vi "UpdateAcquisitionStats.vi"(8 "error in (no error)":errorcluster, 11 "configuration":T1 {"FixedSizeX31"."InputConfig" items=["AC Coupled", "DC Coupled", "IEPE AC Coupled"]}) -> (0 "error out":errorcluster, 2 "settling time requirement met?":bool, 3 "configuration":T1 {"FixedSizeX31"."InputConfig" items=["AC Coupled", "DC Coupled", "IEPE AC Coupled"]})   [LabVIEW 2017, in "McsaFpgaAcquisition.lvlib"]
uses:
  <vilib>/addons/InsightCM/Devices/Shared/Mcsa/McsaFpgaAcquisition/McsaFpgaAcquisition.lvlib
  <vilib>/addons/InsightCM/Devices/Shared/Mcsa/McsaFpgaAcquisition/controls/Configuration.ctl
  <vilib>/addons/InsightCM/Devices/Shared/Cms/CmsAcquisition/controls/FixedSizeArrays.ctl
  <vilib>/LabVIEW Targets/FPGA/cRIO/shared/nicrio_ModuleControls/nicrio_cRIO-9232_ConfigModeRing.ctl
  <vilib>/addons/InsightCM/Devices/Shared/Cms/cRIOWfmAcq/subVIs/RIO Wfm Cust Ctrls/rwfm_SamplingInfo.ctl
  <vilib>/addons/InsightCM/Devices/Shared/Mcsa/McsaFpgaAcquisition/controls/Group.ctl
  <vilib>/addons/InsightCM/Devices/Shared/Mcsa/McsaFpgaAcquisition/controls/ChannelMcsa.ctl
  <vilib>/addons/InsightCM/Devices/Shared/Mcsa/McsaFpgaAcquisition/controls/RangeParams.ctl
  <vilib>/addons/InsightCM/Devices/Shared/Cms/cRIOWfmAcq/cRIOWfmLib.lvlib
  <vilib>/addons/InsightCM/Devices/Shared/Cms/CmsAcquisition/CmsAcquisition.lvlib
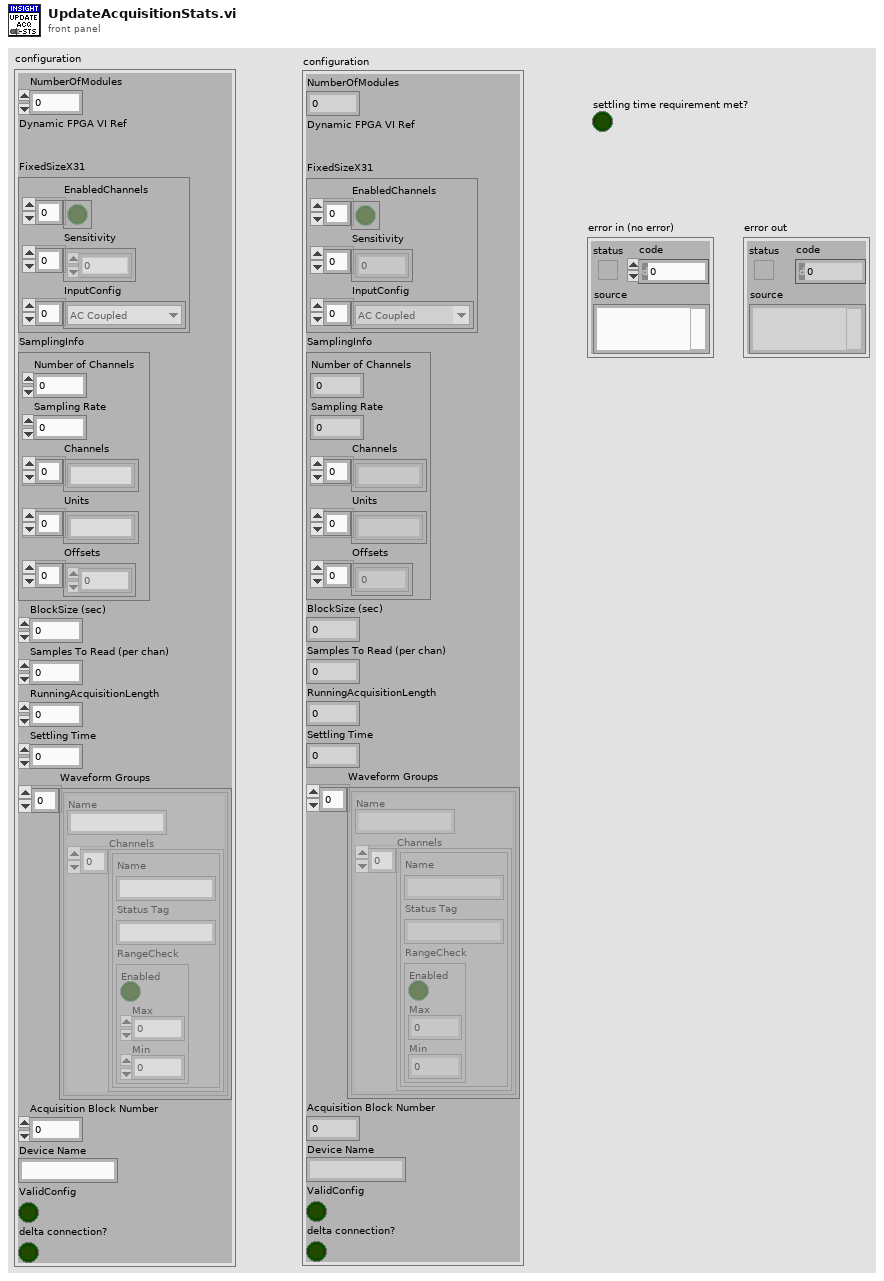
[diagram p1: front panel]
types:
  T1 = typedef "McsaFpgaAcquisition.lvlib/Configuration.ctl" = cluster{"NumberOfModules":i16, "Dynamic FPGA VI Ref":refnum<k20>, "FixedSizeX31":T2, "SamplingInfo":T4, "BlockSize (sec)":dbl, "Samples To Read (per chan)":i32, "RunningAcquisitionLength":dbl, "Settling Time":dbl, "Waveform Groups":T5[], "Acquisition Block Number":i32, "Device Name":string, "ValidConfig":bool, "delta connection?":bool}
  T2 = typedef "CmsAcquisition.lvlib/FixedSizeArrays.ctl" = cluster{"EnabledChannels":bool[], "Sensitivity":dbl[], "InputConfig":T3[]}
  T3 = typedef "nicrio_cRIO-9232_ConfigModeRing.ctl" = u8
  T4 = typedef "cRIOWfmLib.lvlib/rwfm_SamplingInfo.ctl" = cluster{"Number of Channels":i32, "Sampling Rate":dbl, "Channels":string[], "Units":string[], "Offsets":sgl[]}
  T5 = typedef "McsaFpgaAcquisition.lvlib/Group.ctl" = cluster{"Name":string, "Channels":T6[]}
  T6 = typedef "McsaFpgaAcquisition.lvlib/ChannelMcsa.ctl" = cluster{"Name":string, "Status Tag":string, "RangeCheck":T7}
  T7 = typedef "McsaFpgaAcquisition.lvlib/RangeParams.ctl" = cluster{"Enabled":bool, "Max":dbl, "Min":dbl}
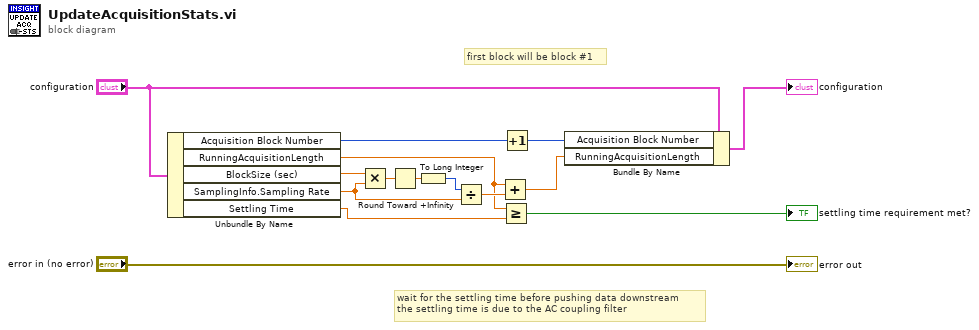
[diagram p0: block diagram]
diagram:
  # "first block will be block #1"
  # "wait for the settling time before pushing data downstream\nthe settling time is due to the AC coupling filter"
  n1 = Unbundle By Name("configuration") -> ("Acquisition Block Number"=w1:i32, "RunningAcquisitionLength"=w8:dbl, "BlockSize (sec)"=w12:dbl, "SamplingInfo.Sampling Rate"=w10:dbl, "Settling Time"=w4:dbl)
  n2 = Multiply(x=w12, y=w10) -> (x*y=w14:dbl)
  n3 = Round Toward +Infinity(x=w14) -> (ceil(x): smallest int >= x=w13:dbl)
  n4 = To Long Integer(number=w13) -> (32bit integer=w11:i32)
  n5 = Divide(x=w11, y=w10) -> (x/y=w15:dbl)
  n6 = Add(x=w8, y=w15) -> (x+y=w3:dbl)
  n7 = Greater Or Equal?(x=w8, y=w4) -> (x >= y?=→"settling time requirement met?":bool)
  n8 = Increment(x=w1) -> (x+1=w2:i32)
  n9 = Bundle By Name(cluster="configuration", "Acquisition Block Number"=w2, "RunningAcquisitionLength"=w3) -> (→"configuration":T1)
  "error out" <- "error in (no error)"
